vi "SetLoadedTools.vi"(8 "error in (no error)":errorcluster caption="entrée d'erreur (pas d'erreur)", 10 "LoadedTools":refnum<class "BaseDevice.lvclass">[](array[class]) caption="LoadedInst", 11 "Experiment en entrée":refnum<class "Experiment.lvclass">) -> (0 "error out":errorcluster caption="sortie d'erreur", 3 "Experiment en sortie":refnum<class "Experiment.lvclass">)   [LabVIEW 2019, in "Experiment.lvclass"]
uses:
  Experiment.lvclass
  DevicesClass/BaseDevice/BaseDevice.lvclass
  Experiment.lvclass/Experiment.ctl
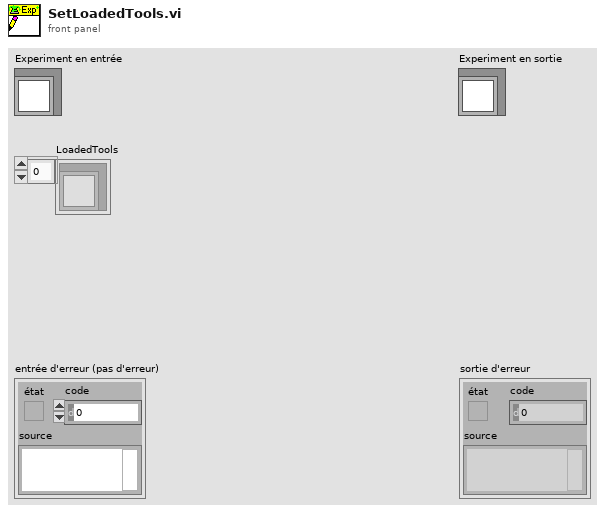
[diagram p1: front panel]
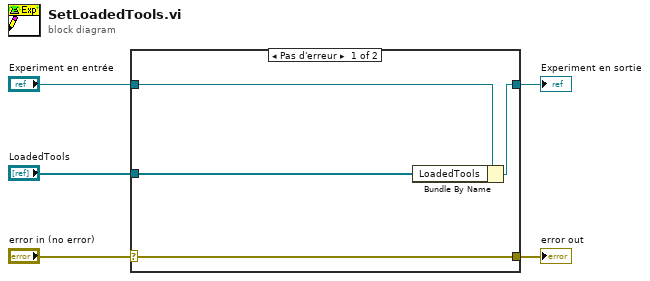
[diagram p0: block diagram]
diagram:
  n1 = case shown="Pas d'erreur" "error in (no error)" {
    selector: "error in (no error)" -> [w9 w10]
    tunnel: [w9 w10] -> w4
    tunnel: [w7 w11] -> w2
    tunnel: "Experiment en entrée" -> [w8 w11]
    tunnel: "LoadedTools" -> [w6 _]
    frame No Error {
      n2 = Bundle By Name(cluster=w8, "LoadedTools"=w6) -> (w7:refnum<class "Experiment.lvclass">)
    }
    frame Error {
    }
  }
  "error out" <- w4
  "Experiment en sortie" <- w2
